vi "CSTK_Icon_Creator_CreateLogo_JudgePath.vi"(8 "error in":errorcluster, 11 "文件夹名输入":string) -> (0 "error out":errorcluster, 2 "result":enum16{"确定", "取消", "重新输入"}(ring), 3 "文件夹路径输出":path)   [LabVIEW 2015, in "CSTK_Icon Creator.lvlib"]
uses:
  CSTK_Icon Creator.lvlib
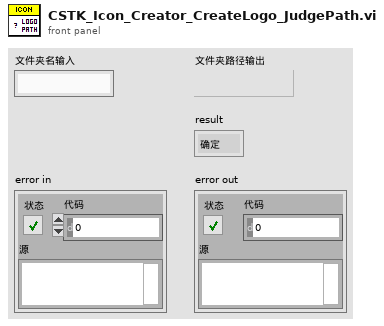
[diagram p1: front panel]
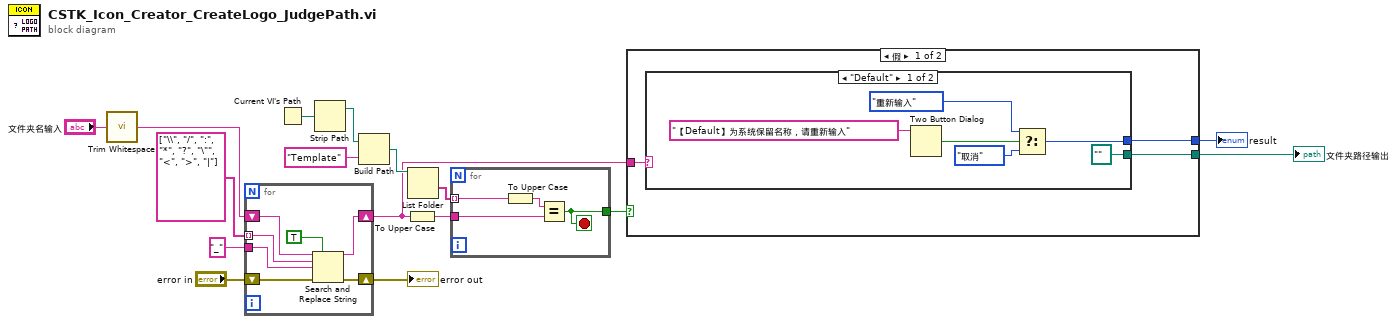
[diagram p0: block diagram]
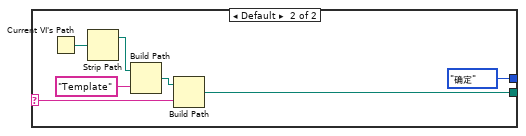
[diagram p2: hidden frame]
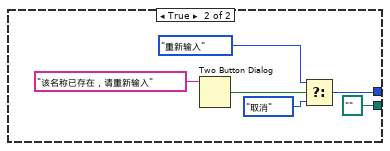
[diagram p3: hidden frame]
diagram:
  n1 = call <vilib>:"Trim Whitespace.vi"("string"="文件夹名输入") -> ("trimmed string"=w9:string)  [unwired: 1 in]
  n2 = for {
    shift-right: [w22] -> w4
    shift-left: w9 -> [w23]
    tunnel: "_" ("替换字符") -> [w21]
    tunnel: string[] ["\\", "/", ":", "*", "?", "\"", "<", ">", "|"] -> [w20] mode=indexing
    shift-right: [w18] -> w1
    shift-left: "error in" -> [w19]
    n3 = Search and Replace String(replace all?=TRUE ("替换全部？(F)"), input string=w23, search string=w20, replace string=w21, error in=w19) -> (result string=w22:string, error out=w18:errorcluster)  [unwired: 3 in, 2 out]
  }
  "error out" <- w1
  n4 = Current VI's Path() -> (path=w14:path)
  n5 = Strip Path(path=w14) -> (stripped path=w15:path)  [unwired: 1 out]
  n6 = Build Path(base path=w15, name or relative path="Template" ("名称或相对路径")) -> (appended path=w13:path)
  n7 = To Upper Case(1:w4) -> (0:w6:string)
  n8 = List Folder(path=w13) -> (folder names=w12:string[])  [unwired: 3 in, 3 out]
  n9 = for {
    tunnel: w12 -> [w27] mode=indexing
    tunnel: w6 -> [w25]
    tunnel: [w24] -> w5
    stop <- w24 stop-if-true
    n10 = To Upper Case(1:w27) -> (0:w26:string)
    n11 = Equal?(x=w26, y=w25) -> (x = y?=w24:bool)
  }
  n12 = case shown="假" w5 {
    tunnel: [w28 path ""] -> w3
    tunnel: w4 -> [w29 _]
    tunnel: [w30 w45] -> w2
    frame False {
      n13 = case shown="\"Default\"" w29 {
        selector: w29 -> [_ w38]
        tunnel: [w31 enum16{"确定", "取消", "重新输入"}."确定" ("result")] -> w30
        tunnel: [path "" ("appended path") w37] -> w28
        frame "Default" {
          n14 = Two Button Dialog(message="【Default】为系统保留名称，请重新输入" ("消息")) -> (T button?=w34:bool)  [unwired: 2 in]
          n15 = Select(t=enum16{"确定", "取消", "重新输入"}."重新输入" ("result"), s=w34, f=enum16{"确定", "取消", "重新输入"}."取消" ("result")) -> (s? t:f=w31:enum16{"确定", "取消", "重新输入"})
        }
        frame Default {
          n16 = Current VI's Path() -> (path=w40:path)
          n17 = Strip Path(path=w40) -> (stripped path=w41:path)  [unwired: 1 out]
          n18 = Build Path(base path=w41, name or relative path="Template" ("名称或相对路径")) -> (appended path=w39:path)
          n19 = Build Path(base path=w39, name or relative path=w38) -> (appended path=w37:path)
        }
      }
    }
    frame True {
      n20 = Two Button Dialog(message="该名称已存在，请重新输入" ("消息")) -> (T button?=w48:bool)  [unwired: 2 in]
      n21 = Select(t=enum16{"确定", "取消", "重新输入"}."重新输入" ("result"), s=w48, f=enum16{"确定", "取消", "重新输入"}."取消" ("result")) -> (s? t:f=w45:enum16{"确定", "取消", "重新输入"})
    }
  }
  "文件夹路径输出" <- w3
  "result" <- w2
